vi "sensitivity  Measurement.vi"(0 "ref in":T5, 1 "测试 类型":string(combo)="VREF", 5 "tasks in":T4, 7 "Waveform Generator":refnum<visa-resource-name>="TCPIP0::192.168.40.72::INSTR", 9 "Data in":variant, 11 "error in (no error)":errorcluster, 12 "Oscilloscope IO":refnum<visa-resource-name>="tcpip0::192.168.40.70::instr") -> (6 "all  data out":T3={"conditions"={"do test?"=TRUE, "test name"="ib trim test", "user test name"="", "temp"=25.0, "spec min 1"=0.0, "spec max 1"=31.0, "spec min 2"=0.0, "spec max 2"=0.0, "spec units"="dec", "type"=enum."absolute", "vin inital"=2.8, "dwell initial"=0.5, "start"=0.0, "stop"=31.0, "step"=1.0, "dwell"=0.2, "bat imp"=0.0, "lead imp"=0.0, "schamber"="a", "gain"=0.0, "spolarity"="t2r", "as"=0.0, "vs"=0.0, "period"=0.0, "pchamber"="a", "ppolarity"="bip\nbip", "aamp"=0.0, "vamp"=0.0, "rchtime"=0.0, "rate"=0.0, "freq"=0.0, "vin end"=0.0, "dwell end"=0.5, "level a"=0.0, "level b"=0.0, "level c"=0.0, "level d"=0.0, "notes"="", "slew time"=25.0, "pw"=0.0, "times"=0.0, "spec min 3"=0.0, "spec max 3"=31.0, "spec min 4"=0.0, "spec max 4"=0.0}, "data out"=[], "result"=[], "TestArrayIndex"=0, "Result Measurement Head"=[]} {"conditions"."spec max 4" format="%^.3e"; "conditions"."spec min 4" format="%^.3e"; "conditions"."spec max 3" format="%^.3e"; "conditions"."spec min 3" format="%^.3e"; "conditions"."times" format="%^.3e"; "conditions"."pw" format="%^.3e"; "conditions"."slew time" format="%.2f"; "conditions"."level a" format="%^.3e"; "conditions"."freq" format="%^.3e"; "conditions"."rate" format="%^.3e"; "conditions"."rchtime" format="%^.3e"; "conditions"."vamp" format="%^.3e"; "conditions"."aamp" format="%^.3e"; "conditions"."period" format="%^.3e"; "conditions"."vs" format="%^.3e"; "conditions"."as" format="%^.3e"; "conditions"."gain" format="%^.3e"; "conditions"."lead imp" format="%^.3e"; "conditions"."bat imp" format="%^.3e"; "conditions"."spec max 2" format="%^.3e"; "conditions"."spec min 2" format="%^.3e"; "conditions"."level d" format="%^.3e"; "conditions"."level c" format="%^.3e"; "conditions"."level b" format="%^.3e"; "conditions"."dwell end" format="%^.3e"; "conditions"."vin end" format="%^.3e"; "conditions"."dwell" format="%^.3e"; "conditions"."step" format="%^.3e"; "conditions"."stop" format="%^.3e"; "conditions"."start" format="%^.3e"; "conditions"."dwell initial" format="%^.3e"; "conditions"."vin inital" format="%^.3e"; "conditions"."spec max 1" format="%^.3e"; "conditions"."spec min 1" format="%^.3e"; "conditions"."temp" format="%.2f"}, 10 "Measurement":string[](array[string]), 15 "Waveform Graph Cal":waveform(dbl)(graph))   [LabVIEW 2016]
uses:
  AET/TypeDef/Pacemaker ASIC Test_Reference.ctl
  AET/TypeDef/Pacemaker ASIC Test_Task.ctl
  AET/TypeDef/Pacemaker ASIC Test_Condition.ctl
  AET/TypeDef/Pacemaker ASIC Test_Register Mark Type.ctl
  Global Variables/Pacemaker ASIC Test_Save_SN Globals.vi
panel:
  in  "Pace Rate":string="60"
  in  "Frquency":dbl=66.76 format="%#_13g"
  in  "offset with pace interval(s)":dbl=0.06 format="%#_13g"
  in  "Phase":dbl=-24.0 format="%#_13g"
  in  "Symmetry":dbl=13.0 format="%#_13g"
  in  "Power ON/off":bool=TRUE
  in  "Burst ON/off":bool=TRUE
  in  "Waveform":T1(ring)
  in  "Amp(vpp)":dbl=0.002 format="%#_13g"
  out "Save_SN":path
  out "Pass/Fail":bool
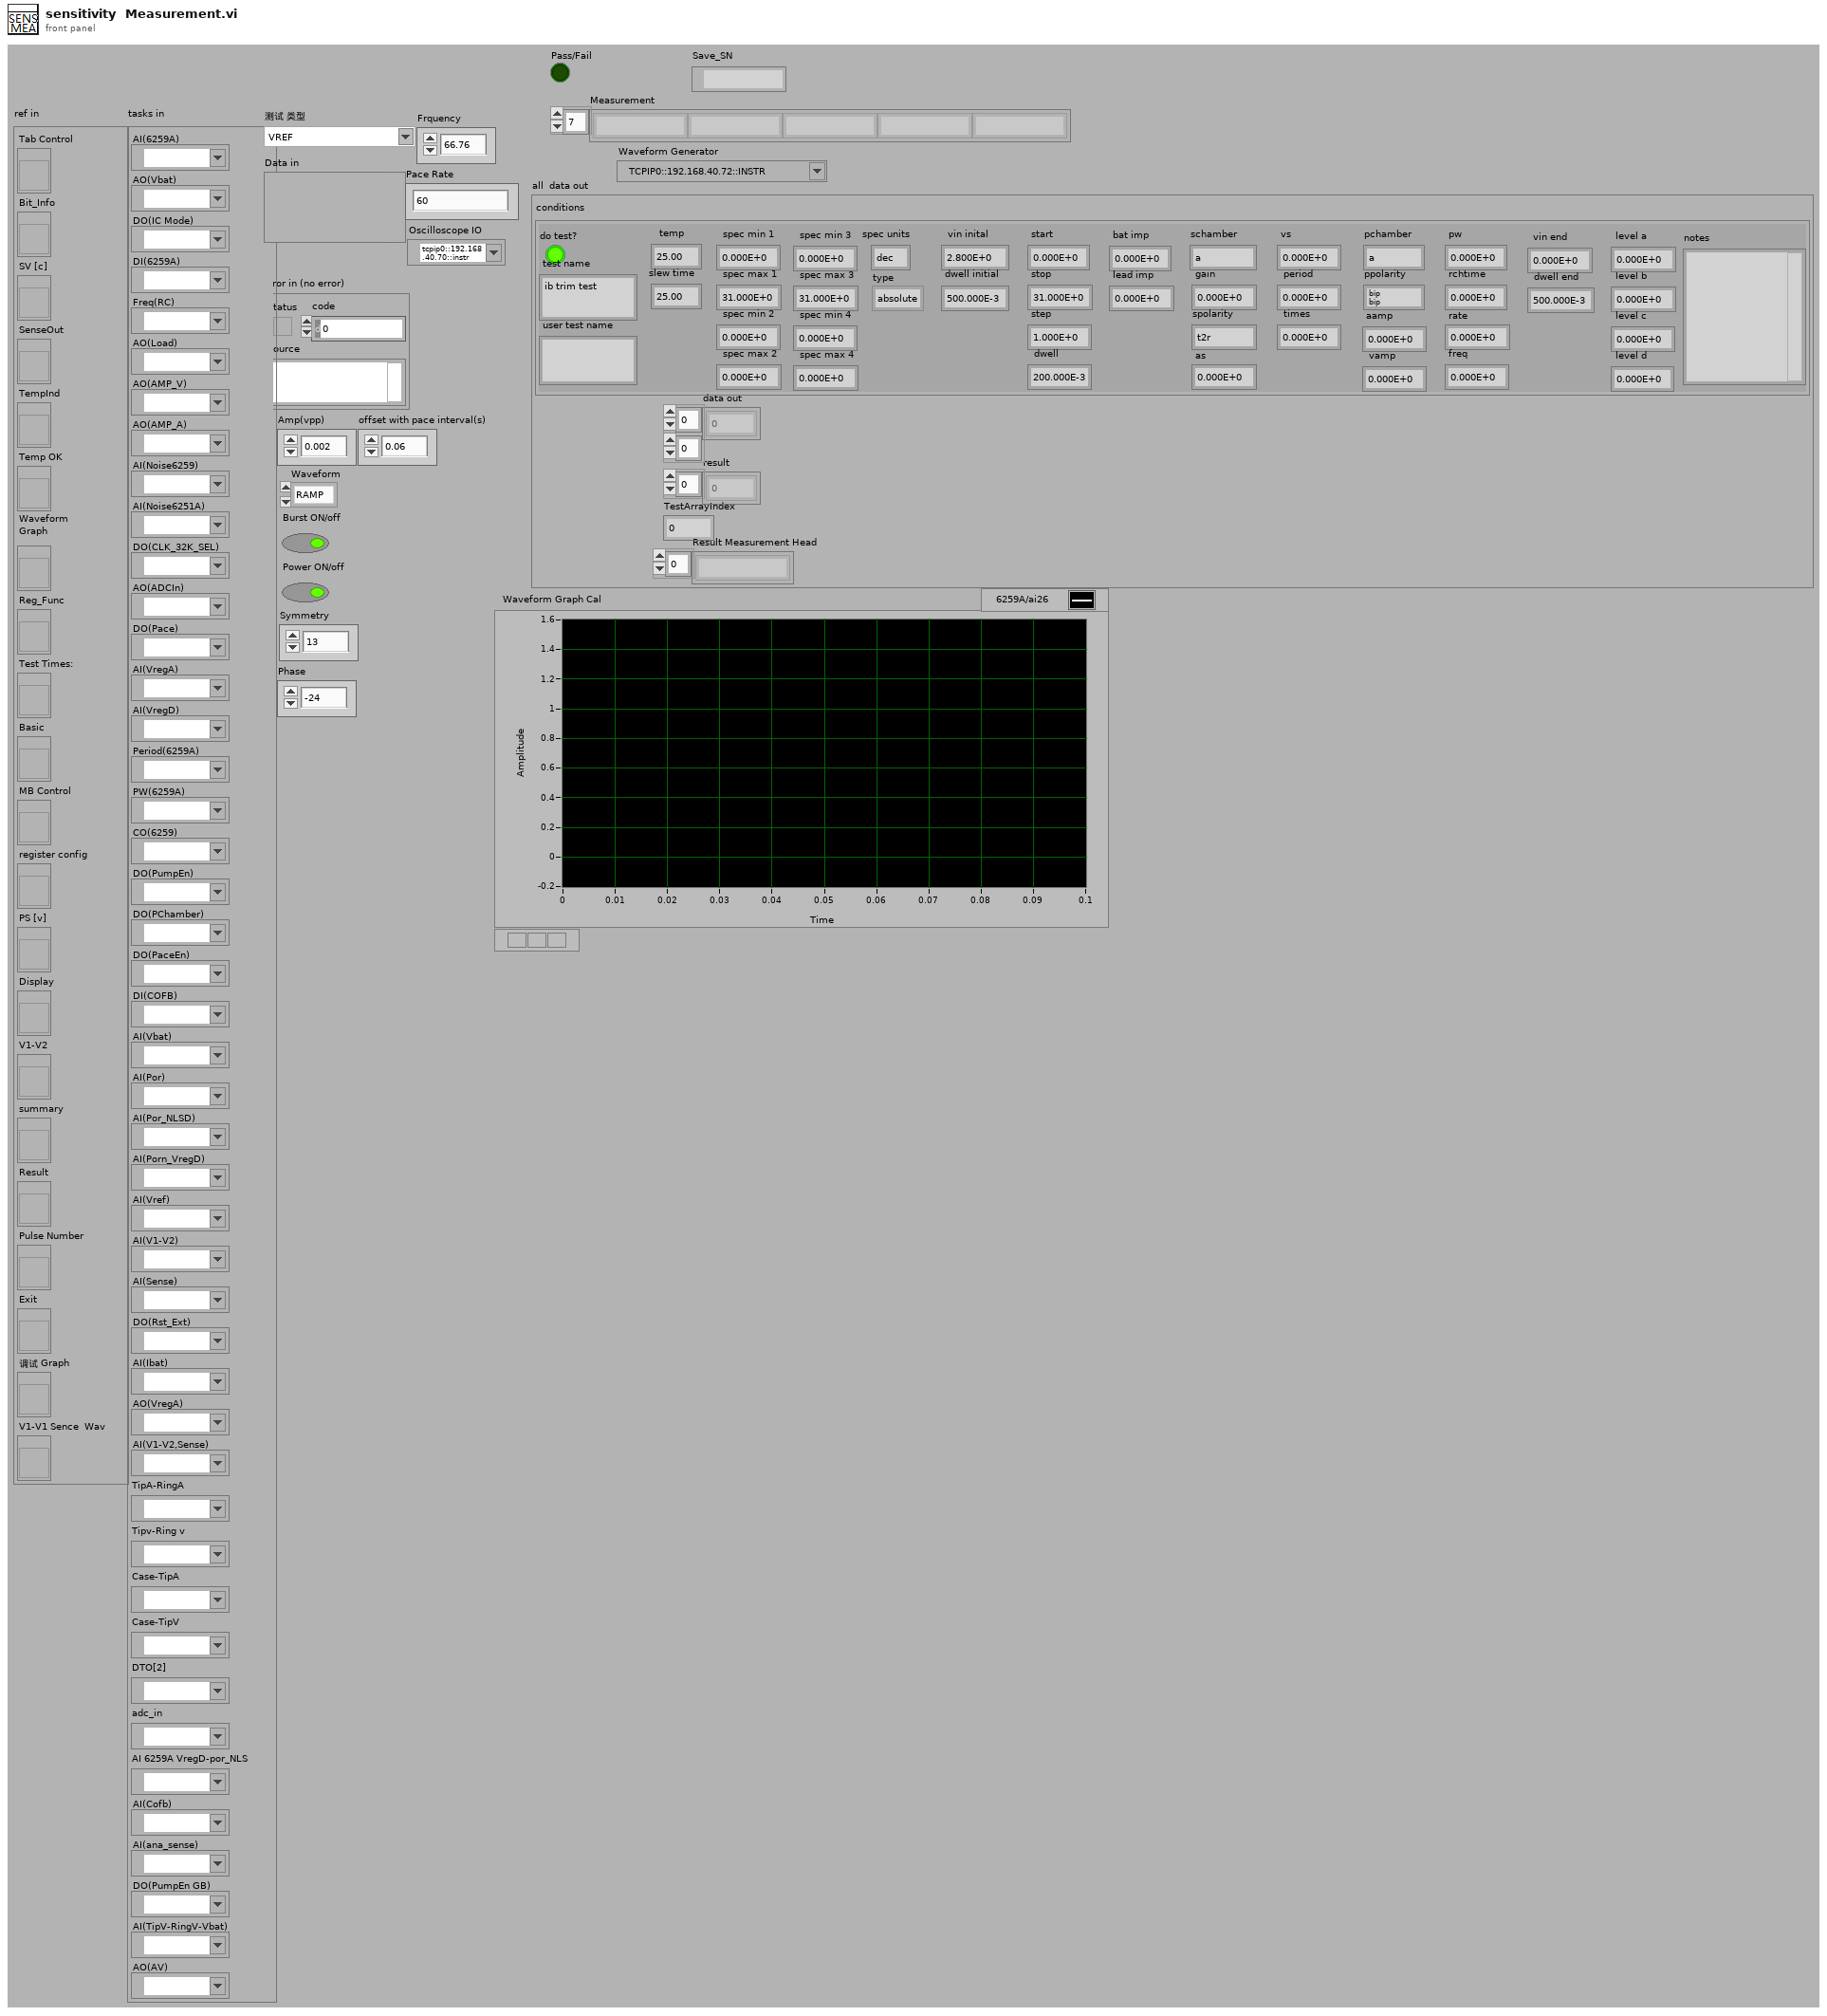
[diagram p1: front panel]
types:
  T1 = enum16{"RAMP", "SINusoid", "SQUare", "TRIangle", "PULSe", "PRBS", "ARB", "DC", "NOISe"}
  T2 = typedef "Pacemaker ASIC Test_Condition.ctl" = cluster{"do test?":bool, "test name":string, "user test name":string, "temp":dbl, "spec min 1":dbl, "spec max 1":dbl, "spec min 2":dbl, "spec max 2":dbl, "spec units":string, "type":enum16{"absolute", "v change", "pct change"}, "vin inital":dbl, "dwell initial":dbl, "start":dbl, "stop":dbl, "step":dbl, "dwell":dbl, "bat imp":dbl, "lead imp":dbl, "schamber":string, "gain":dbl, "spolarity":string, "as":dbl, "vs":dbl, "period":dbl, "pchamber":string, "ppolarity":string, "aamp":dbl, "vamp":dbl, "rchtime":dbl, "rate":dbl, "freq":dbl, "vin end":dbl, "dwell end":dbl, "level a":dbl, "level b":dbl, "level c":dbl, "level d":dbl, "notes":string, "slew time":dbl, "pw":dbl, "times":dbl, "spec min 3":dbl, "spec max 3":dbl, "spec min 4":dbl, "spec max 4":dbl}
  T3 = cluster{"conditions":T2, "data out":dbl[][], "result":dbl[], "TestArrayIndex":i32, "Result Measurement Head":string[]}
  T4 = typedef "Pacemaker ASIC Test_Task.ctl" = cluster{"AI(6259A)":refnum<k21>, "AO(Vbat)":refnum<k21>, "DO(IC Mode)":refnum<k21>, "DI(6259A)":refnum<k21>, "Freq(RC)":refnum<k21>, "AO(Load)":refnum<k21>, "AO(AMP_V)":refnum<k21>, "AO(AMP_A)":refnum<k21>, "AI(Noise6259)":refnum<k21>, "AI(Noise6251A)":refnum<k21>, "DO(CLK_32K_SEL)":refnum<k21>, "AO(ADCIn)":refnum<k21>, "DO(Pace)":refnum<k21>, "AI(VregA)":refnum<k21>, "AI(VregD)":refnum<k21>, "Period(6259A)":refnum<k21>, "PW(6259A)":refnum<k21>, "CO(6259)":refnum<k21>, "DO(PumpEn)":refnum<k21>, "DO(PChamber)":refnum<k21>, "DO(PaceEn)":refnum<k21>, "DI(COFB)":refnum<k21>, "AI(Vbat)":refnum<k21>, "AI(Por)":refnum<k21>, "AI(Por_NLSD)":refnum<k21>, "AI(Porn_VregD)":refnum<k21>, "AI(Vref)":refnum<k21>, "AI(V1-V2)":refnum<k21>, "AI(Sense)":refnum<k21>, "DO(Rst_Ext)":refnum<k21>, "AI(Ibat)":refnum<k21>, "AO(VregA)":refnum<k21>, "AI(V1-V2,Sense)":refnum<k21>, " TipA-RingA":refnum<k21>, "Tipv-Ring v":refnum<k21>, " Case-TipA":refnum<k21>, "Case-TipV":refnum<k21>, "DTO[2]":refnum<k21>, "adc_in":refnum<k21>, "AI 6259A VregD-por_NLS":refnum<k21>, "AI(Cofb)":refnum<k21>, "AI(ana_sense)":refnum<k21>, "DO(PumpEn GB)":refnum<k21>, "AI(TipV-RingV-Vbat)":refnum<k21>, "AO(AV)":refnum<k21>}
  T5 = typedef "Pacemaker ASIC Test_Reference.ctl" = cluster{"Tab Control":refnum<vi>, "Bit_Info":refnum<vi>, "SV [c]":refnum<vi>, "SenseOut":refnum<vi>, "TempInd":refnum<vi>, "Temp OK":refnum<vi>, "Waveform \nGraph":refnum<vi>, "Reg_Func":refnum<vi>, "Test Times:":refnum<vi>, "Basic":refnum<vi>, "MB Control":refnum<vi>, "register config":refnum<vi>, "PS [v]":refnum<vi>, "Display":refnum<vi>, "V1-V2":refnum<vi>, "summary":refnum<vi>, "Result":refnum<vi>, "Pulse Number":refnum<vi>, "Exit":refnum<vi>, "调试 Graph":refnum<vi>, "V1-V1 Sence  Wav ":refnum<vi>}
  T6 = typedef "Pacemaker ASIC Test_Register Mark Type.ctl" = enum16{"no action", "TRIM_BANDGAPV", "TRIM_VREGD", "TRIM_VREGA", "TRIM_IBIAS", "TRIM_HPFBW", "TRIM_LPFBW", "TRIM_RC32k", "TRIM_RC1p6k", "TRIM_IBIPT_A", "TRIM_IBIPT_V", "ASGN", "AS", "AUR_UT", "APAMP", "APW", "APUMPGN", "ARCHG", "ABILUNISEL", "VSGN", "VS", "VUR_UT", "VPAMP", "VPW", "VPUMPGN", "VRCHG", "VBILUNISEL", "Test_sel_a", "Test_sel_b", "DTO_SEL", "FBCMEN", "CPEN", "RC1p6kEN", "AntDTM", "ANTENN", "EGMFS REQ", "RC32kEN", "CPUOK", "ENOBLP1", "ENOBLP2", "OBLANK", "PDSA1", "PDSV1", "CSAEN", "CSVEN", "BIR RL", "BIR RH", "MREQ", "RK_SEL", "MRESULT1", "MRESULT2", "TrimOTA_0S1", "TrimOTA_0S2", "TrimOTV_0S1", "TrimOTV_0S2", "ENCASES", "TRIM_HPFBW_H_A", "TRIM_HPFBW_L_A", "TRIM_LPFBW_A", "TRIM_HPFBW_H_V", "TRIM_HPFBW_L_V", "TRIM_LPFBW_V", "R_C_Sel", "PDCHG", "ASIC VVI"}
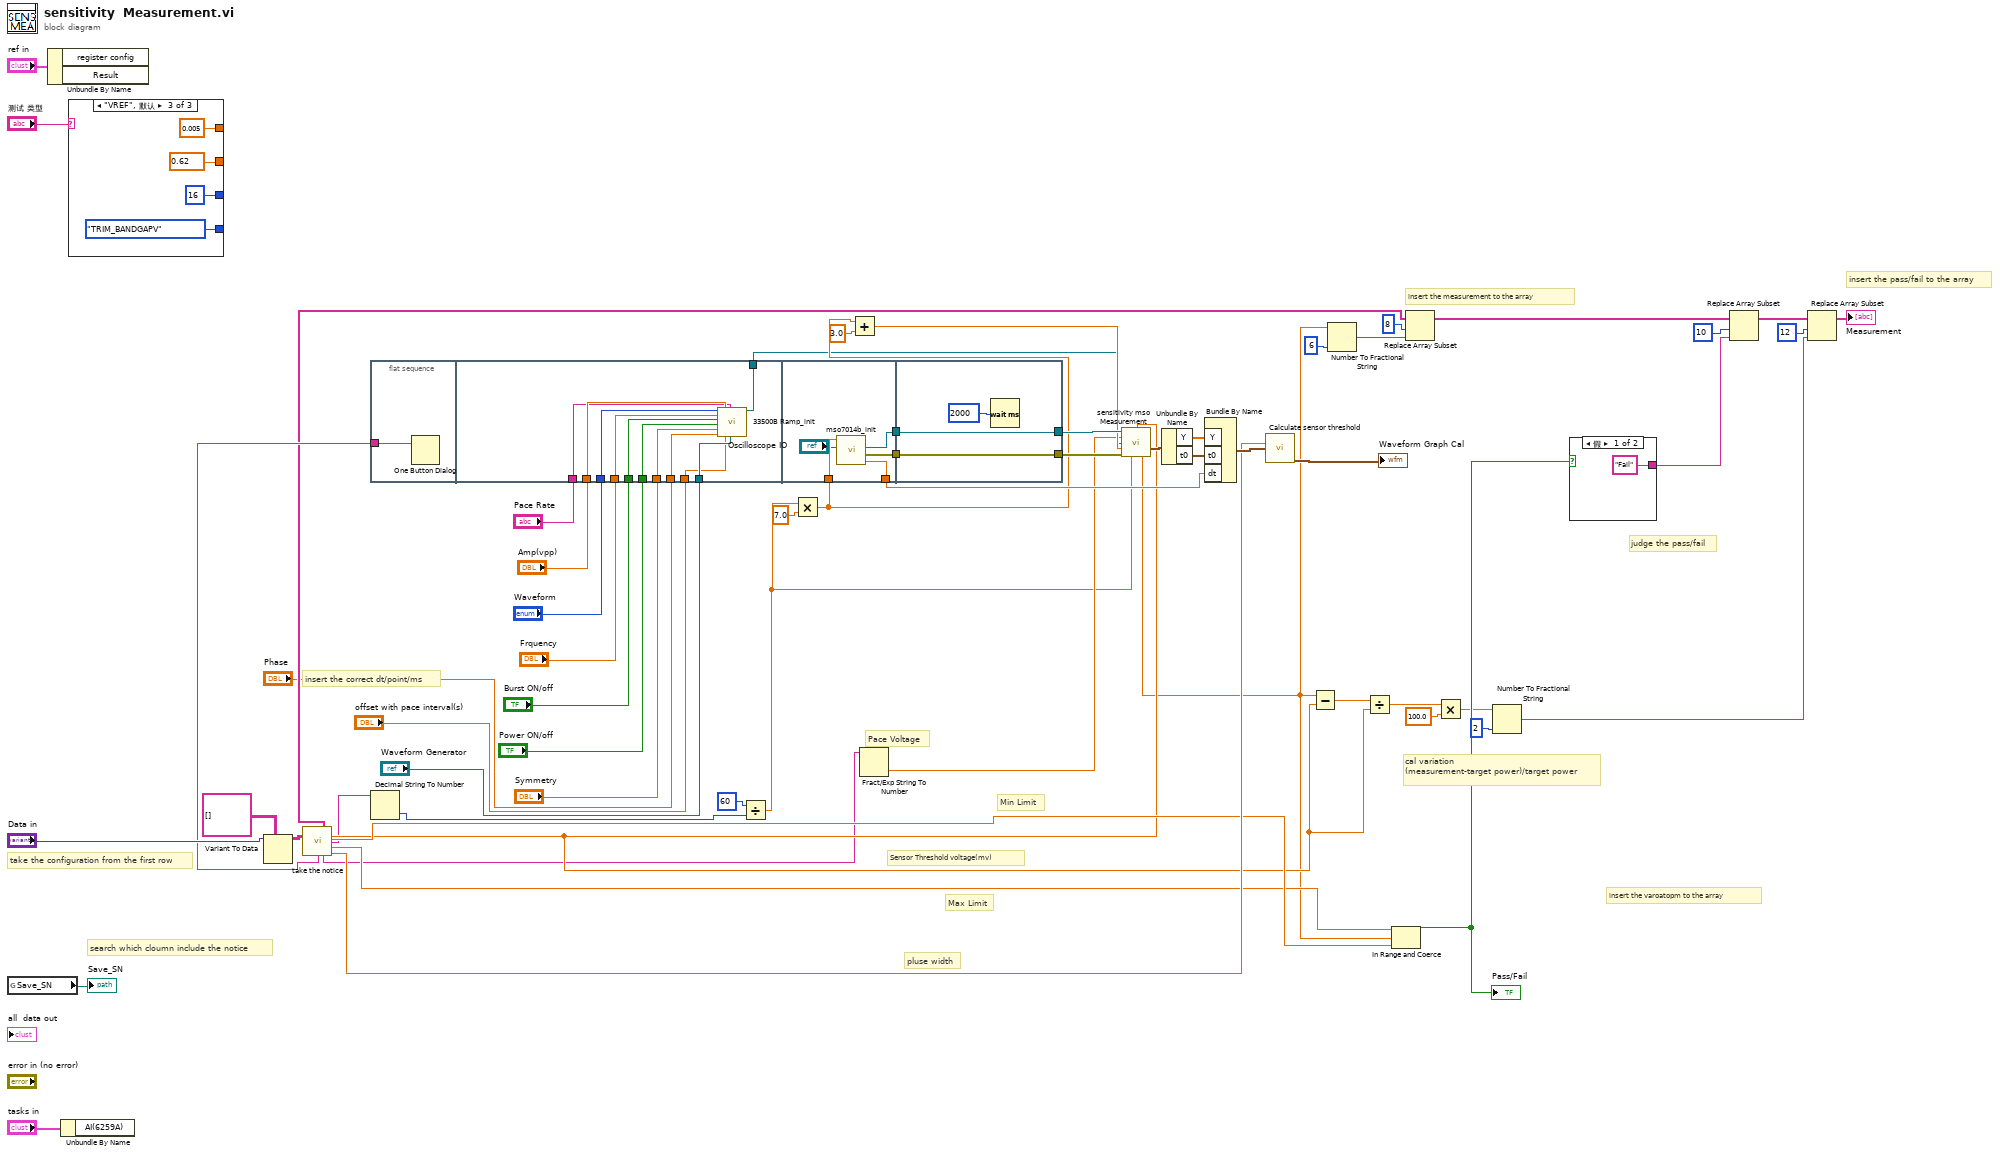
[diagram p0: block diagram]
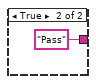
[diagram p2: hidden frame]
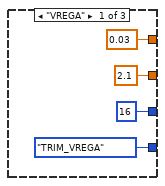
[diagram p3: hidden frame]
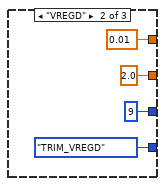
[diagram p4: hidden frame]
diagram:
  # "Pace Voltage"
  # "pluse width"
  # "insert the correct dt/point/ms"
  # "take the configuration from the first row"
  # "search which cloumn include the notice"
  # "insert the pass/fail to the array"
  # "insert the varoatopm to the array"
  # "insert the measurement to the array"
  # "judge the pass/fail"
  # "cal variation\n(measurement-target power)/target power"
  # "Sensor Threshold voltage(mv)"
  # "Min Limit"
  # "Max Limit"
  n1 = global read "Pacemaker ASIC Test_Save_SN Globals.vi" "Save_SN"() -> (→"Save_SN":path)
  n2 = Unbundle By Name("ref in") -> ()  [unwired: 2 out]
  n3 = Unbundle By Name("tasks in") -> ()  [unwired: 1 out]
  n4 = case shown="\"VREF\", 默认" "测试 类型" {
    tunnel: [Pacemaker_ASIC_Test_Register_Mark_Type."TRIM_VREGA" ("Reg Mark") Pacemaker_ASIC_Test_Register_Mark_Type."TRIM_VREGD" ("Reg Mark") Pacemaker_ASIC_Test_Register_Mark_Type."TRIM_BANDGAPV" ("Reg Mark")] -> _
    tunnel: [2.1 ("y") 2.0 ("y") 0.62 ("y")] -> _
    tunnel: [u8 16 ("y") u8 9 ("y") u8 16 ("y")] -> _
    tunnel: [0.03 ("y") 0.01 ("y") 0.005 ("y")] -> _
    frame "VREGA" {
    }
    frame "VREGD" {
    }
    frame "VREF", Default {
    }
  }
  n5 = Variant To Data(type=string[][] [], Variant="Data in") -> (data=w24:string[][])  [unwired: 1 in, 1 out]
  n6 = call "take the notice.vi"("数组"=w24) -> ("Original array"=w25:string[], "Target"=w7:dbl, "Min"=w28:dbl, "Pace Rate"=w5:string, "Max"=w27:dbl, "notice"=w26:string, "pace amp"=w4:string, "Pluse Width"=w29:dbl)  [unwired: 7 in]
  n7 = flat-sequence {
    tunnel: w26 -> [w74]
    tunnel: "Waveform Generator" -> [w85]
    tunnel: "Frquency" -> [w84]
    tunnel: "Amp(vpp)" -> [w83]
    tunnel: "Waveform" -> [w82]
    tunnel: "Burst ON/off" -> [w81]
    tunnel: "Power ON/off" -> [w80]
    tunnel: "Symmetry" -> [w79]
    tunnel: "Phase" -> [w78]
    tunnel: "offset with pace interval(s)" -> [w77]
    tunnel: "Pace Rate" -> [w76]
    tunnel: [w75] -> w1
    tunnel: [w90] -> w51
    tunnel: [w89] -> w50
    tunnel: [w88] -> w43
    tunnel: w11 -> [w87]
    tunnel: [w92] -> w55
    tunnel: [w93] -> w56
    tunnel: w51 -> [w93]
    tunnel: w50 -> [w92]
    frame #0 {
      n8 = One Button Dialog(message=w74) -> ()  [unwired: 1 in, 1 out]
    }
    frame #1 {
      n9 = call "33500B Ramp_init.vi"("Waveform"=w82, "Frquency"=w84, "Burst ON/off"=w81, "Power ON/off"=w80, "Symmetry"=w79, "Phase"=w78, "Amp(vpp)"=w83, "offset with pace interval(s)"=w77, "Pace Rate"=w76, "VISA资源名称"=w85) -> ("VISA资源名称输出"=w75:refnum<visa-resource-name>)  [unwired: 9 in]
    }
    frame #2 {
      n10 = call "mso7014b_init.vi"("Oscilloscope IO"="Oscilloscope IO", "Timebase (20.0E-9)"=w87) -> ("dt"=w88:dbl, "error out"=w89:errorcluster, "VISA resource name out"=w90:refnum<visa-resource-name>)  [unwired: 7 in]
    }
    frame #3 {
      n11 = Wait (ms)(milliseconds to wait=u32 2000 ("等待时间（毫秒）")) -> ()  [unwired: 1 out]
    }
  }
  n12 = Decimal String To Number(string=w5) -> (number=w3:i32)  [unwired: 2 in, 1 out]
  n13 = Divide(x=60, y=w3) -> (x/y=w2:dbl)
  n14 = Multiply(x=w2, y=7.0) -> (x*y=w11:dbl)
  n15 = Add(x=w11, y=3.0) -> (x+y=w9:dbl)
  n16 = Fract/Exp String To Number(string=w4) -> (number=w8:dbl)  [unwired: 3 in, 1 out]
  n17 = call "sensitivity mso Measurement.vi"("OSC"=w56, "Sensor Threshold Setting"=w7, "Pace Voltage"=w8, "Waveform Generator"=w1, "Delay"=w9, "error in (no error)"=w55, "Pace interval"=w2) -> ("CH1 Waveform"=w42:waveform(dbl), "Sensor Threshold"=w6:dbl)  [unwired: 5 in, 2 out]
  n18 = Unbundle By Name(w42) -> ("Y"=w45:dbl[], "t0"=w44:timestamp)
  n19 = Bundle By Name("Y"=w45, "t0"=w44, "dt"=w43) -> (w41:waveform(dbl))  [unwired: 1 in]
  n20 = call "Calculate sensor threshold.vi"("设定脉宽"=w29, "Test Result"=w41) -> ("Waveform Graph Cal"=→"Waveform Graph Cal":waveform(dbl))  [unwired: 4 in, 9 out]
  n21 = Subtract(x=w6, y=w7) -> (x-y=w38:dbl)
  n22 = Number To Fractional String(number=w6, precision (6)=i16 6 ("精度(6)")) -> (F-format string=w53:string)  [unwired: 2 in]
  n23 = Divide(x=w38, y=w7) -> (x/y=w37:dbl)
  n24 = In Range and Coerce(upper limit=w27, x=w6, lower limit=w28) -> (In Range?=w49:bool)  [unwired: 1 out]
  "Pass/Fail" <- w49
  n25 = Replace Array Subset(array=w25, new element=w53, index=8 ("索引")) -> (w39:string[])
  n26 = Multiply(x=w37, y=100.0) -> (x*y=w34:dbl)
  n27 = Number To Fractional String(number=w34, precision (6)=i16 2 ("精度(6)")) -> (F-format string=w32:string)  [unwired: 2 in]
  n28 = case shown="假" w49 {
    tunnel: ["Fail" "Pass"] -> w48
    frame False {
    }
    frame True {
    }
  }
  n29 = Replace Array Subset(array=w39, new element=w48, index=10 ("索引")) -> (w35:string[])
  n30 = Replace Array Subset(array=w35, new element=w32, index=12 ("索引")) -> (→"Measurement":string[])
